vi "Process.vi"(8 "error in":errorcluster, 11 "Pump":refnum<class "Pump.lvclass">) -> (0 "error out":errorcluster, 3 "Pump out":refnum<class "Pump.lvclass">)   [LabVIEW 2014, in "Pump.lvclass"]
doc: "JKI State Machine Objects (SMO) 1.4.0.57\nJKI - JKI\nCopyright (c) 2018, JKI"
uses:
  Pump.lvclass
  <vilib>/JKI/JKI SMO/SMO/Typedefs/Parent Call--Enum.ctl
  Pump.lvclass/Pump.ctl
  Pump State - cluster.ctl
  <vilib>/addons/control/pid/pid.llb/PID Advanced (DBL).vi
  <vilib>/JKI/JKI SMO/SMO/SMO.lvclass
  <vilib>/addons/control/pid/NI_PID_pid.lvlib
panel:
  out "Pump State":T1(graph)
  # "For instructions on how to use the JKI State Machine Objects, examples and video tutorials, visit:\nhttp://jki.net/state-machine-objects/\n\nJKI State Machine Objects™\nhttp://jki.net/state-machine-objects/\nCopyright (C) 2005-2015, JKI <info@jki.net>\nALL RIGHTS RESERVED"
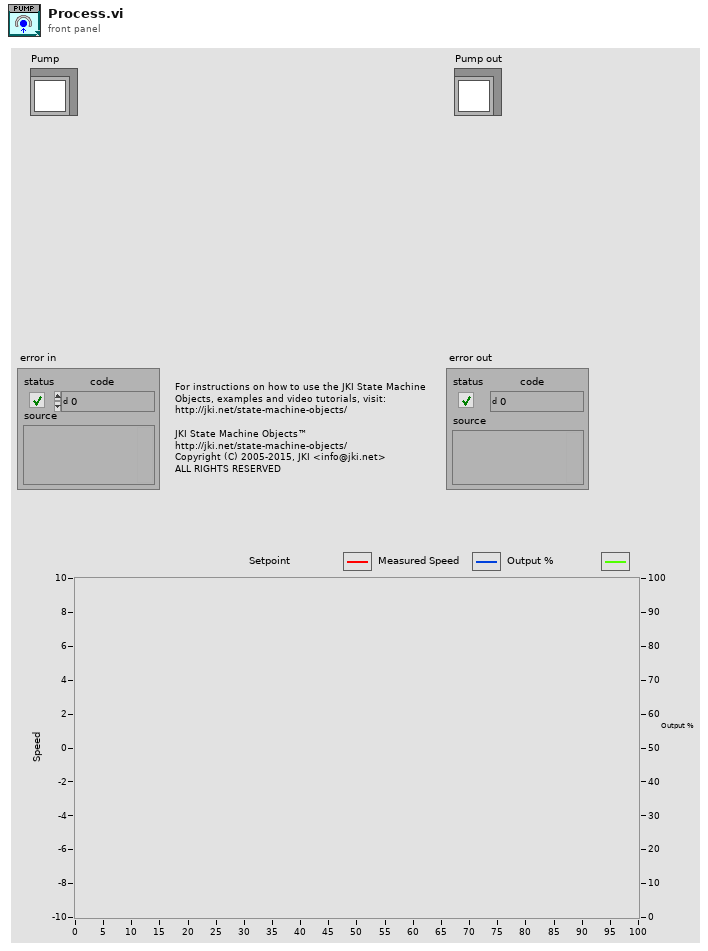
[diagram p1: front panel]
types:
  T1 = typedef "Pump.lvclass/Pump State - cluster.ctl" = cluster{"Pump Setpoint":dbl, "Pump Speed":dbl, "Output %":dbl}
  T2 = typedef "SMO.lvclass/Parent Call--Enum.ctl" = enum16{"Allows parent to run", "Does not request parent to run"}
  T3 = enum32{"invalid app kind", "Development System", "Run Time System", "Student Edition", "Embedded LabVIEW", "Evaluation", "Custom"}
  T4 = enum32{"Invalid", "Standard", "Closed", "Hidden", "Minimized", "Maximized"}
  T5 = cluster{"proportional gain (Kc)":dbl, "integral time (Ti, min)":dbl, "derivative time (Td, min)":dbl}
  T6 = typedef "Pump.lvclass/Parameters - cluster.ctl" = cluster{"Kc":dbl, "Ti":dbl, "Td":dbl, "Min Speed":dbl, "Max Speed":dbl}
  T7 = cluster{"Core":cluster{"Current VI Reference":refnum<vi>, "Close Panel on Exit?":bool, "error":errorcluster}, "Self Reference":refnum<class "Pump.lvclass">, "Parameters":T6, "Speed":dbl}
  T8 = cluster{"Current VI Reference":refnum<vi>, "Close Panel on Exit?":bool, "error":errorcluster}
  T9 = typedef "SMO.lvclass/Protected Events.ctl" = cluster{"StopProcesses":refnum<user-event>, "AbortProcesses":refnum<user-event>, "Config Changed":refnum<user-event>, "Dependency":refnum<user-event>}
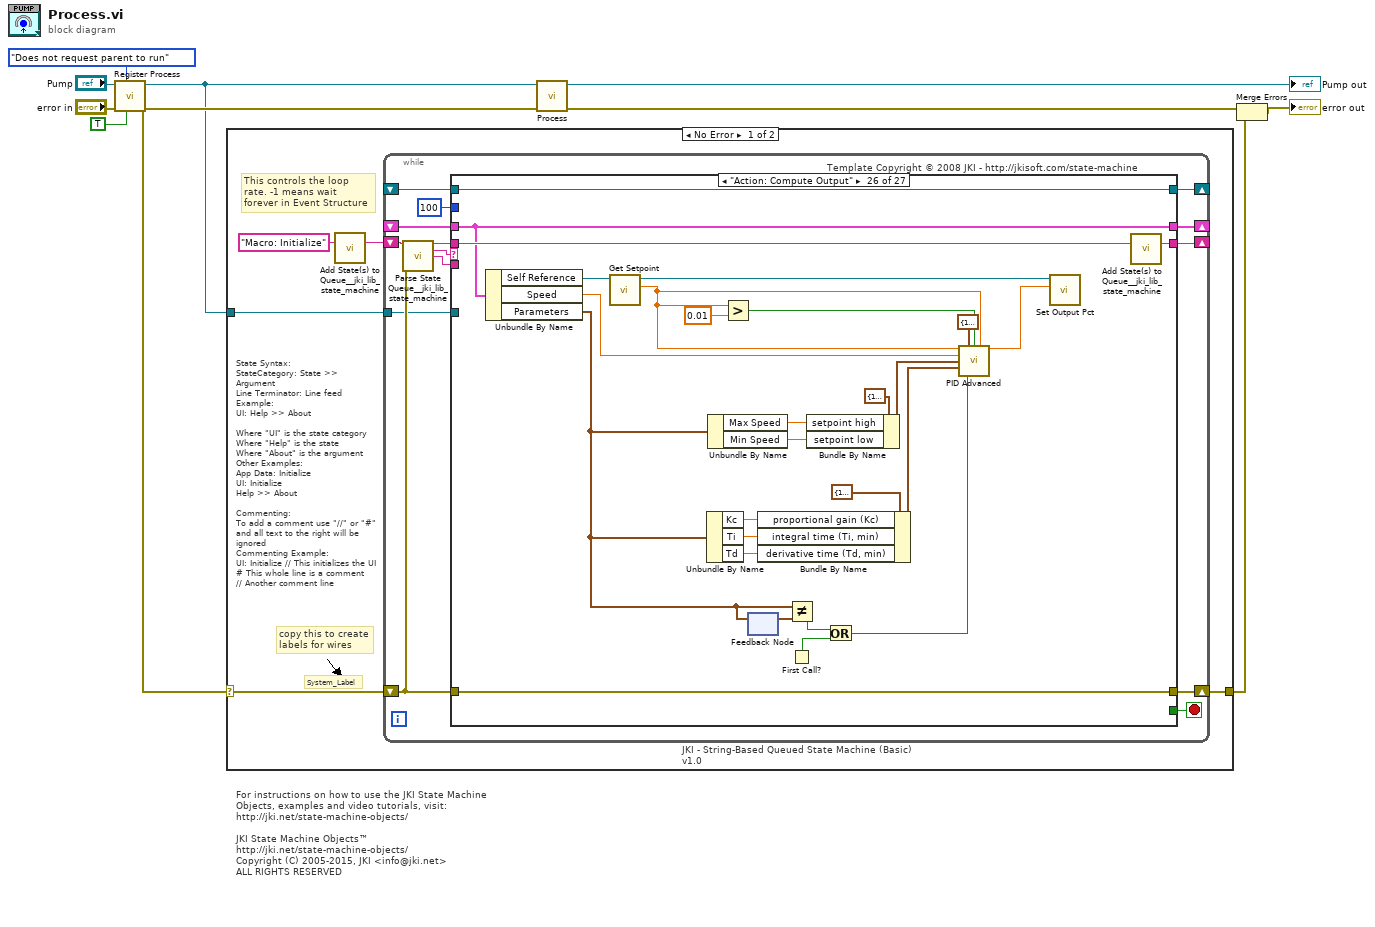
[diagram p0: block diagram]
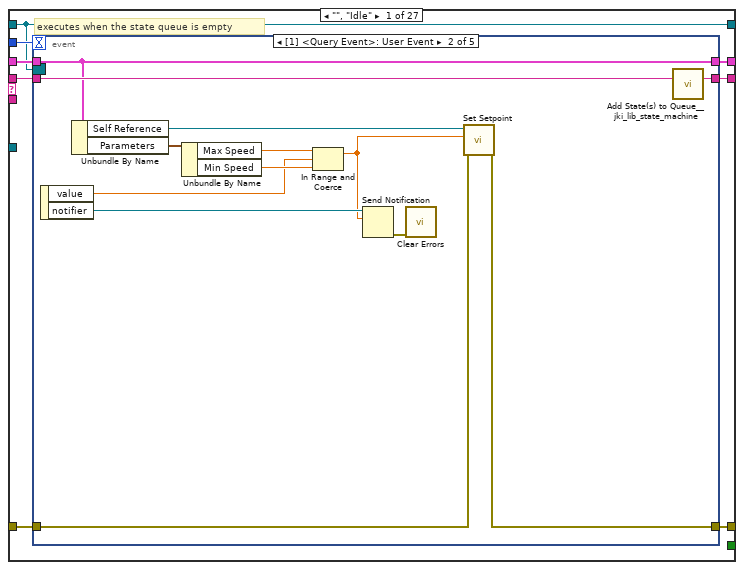
[diagram p2: hidden frame]
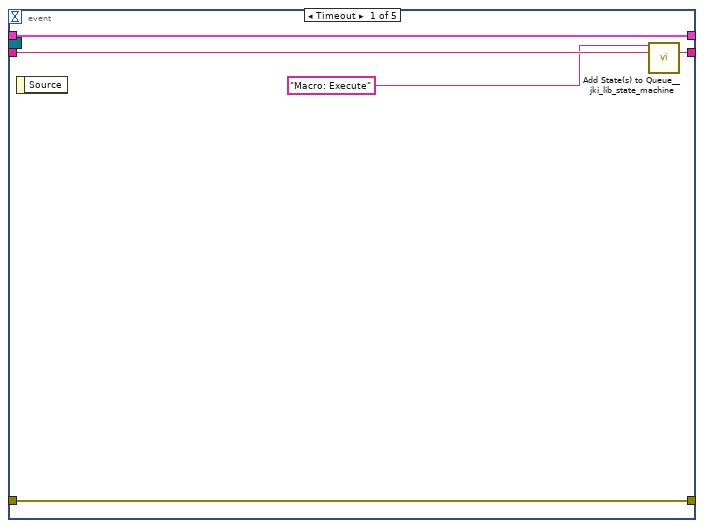
[diagram p3: hidden frame]
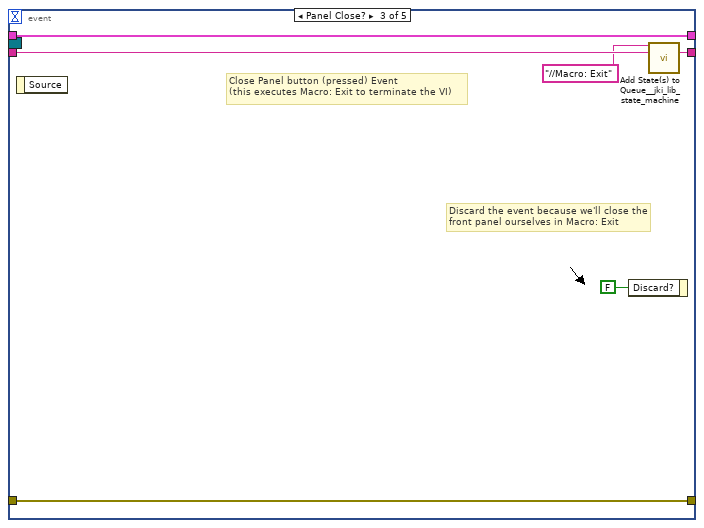
[diagram p4: hidden frame]
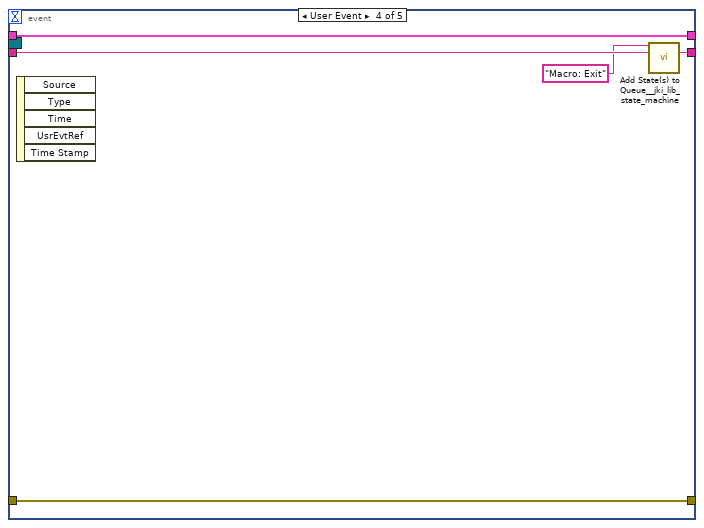
[diagram p5: hidden frame]
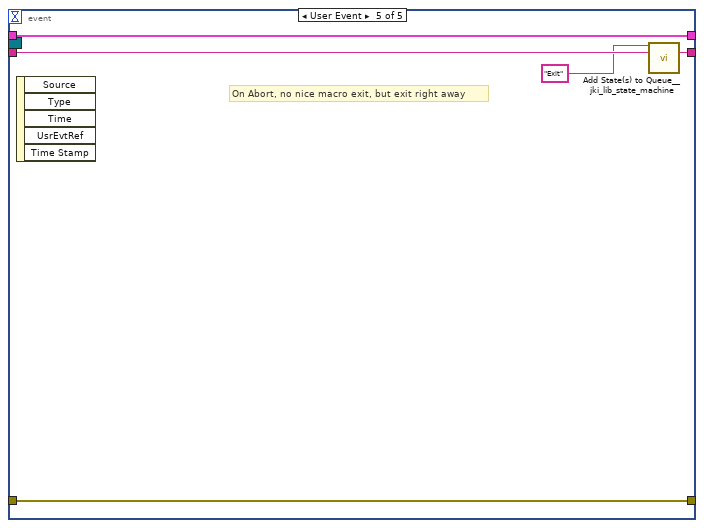
[diagram p6: hidden frame]
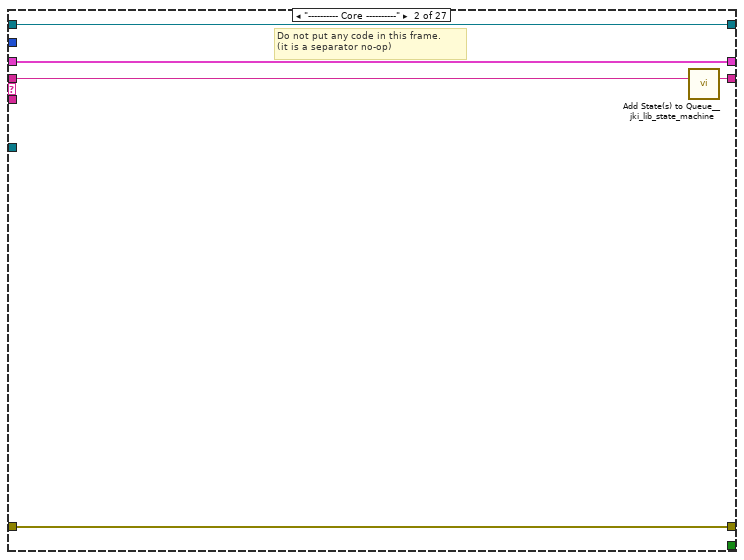
[diagram p7: hidden frame]
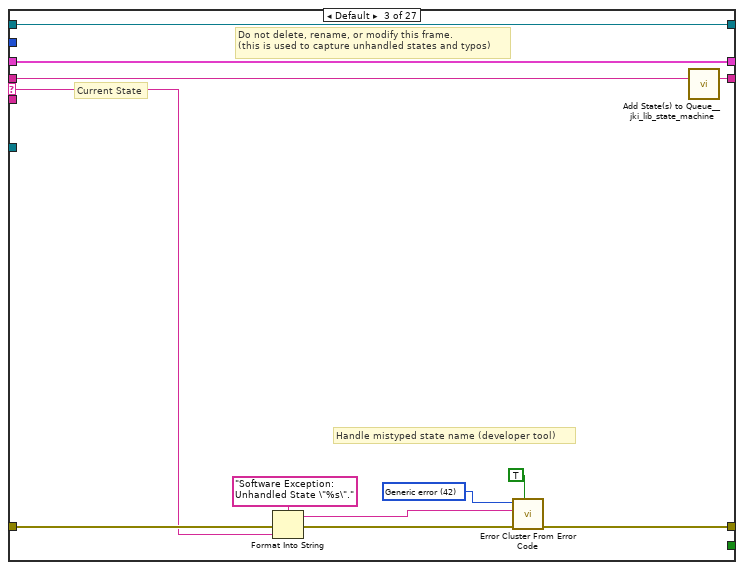
[diagram p8: hidden frame]
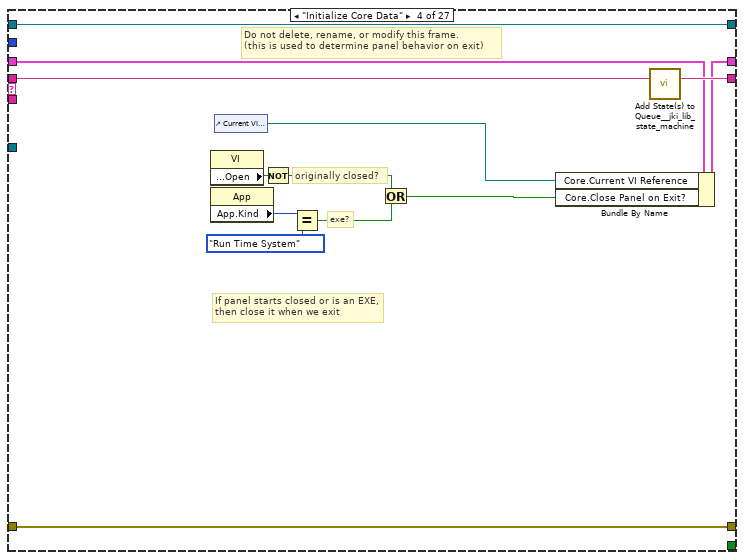
[diagram p9: hidden frame]
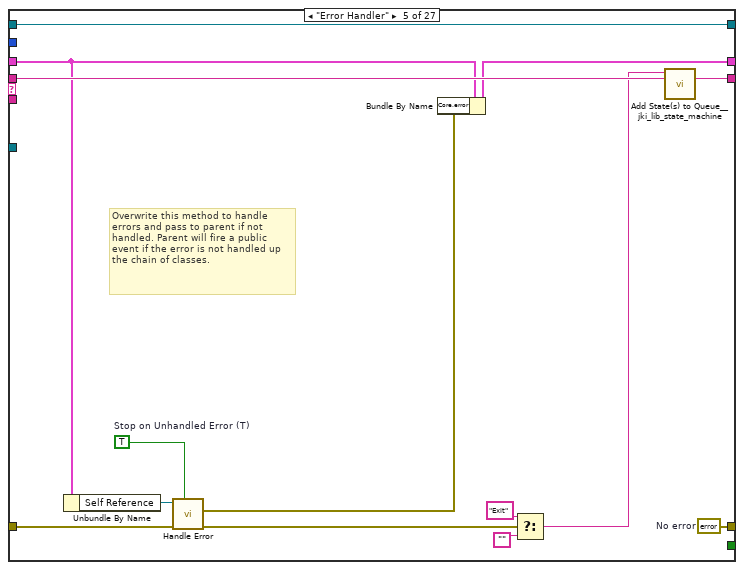
[diagram p10: hidden frame]
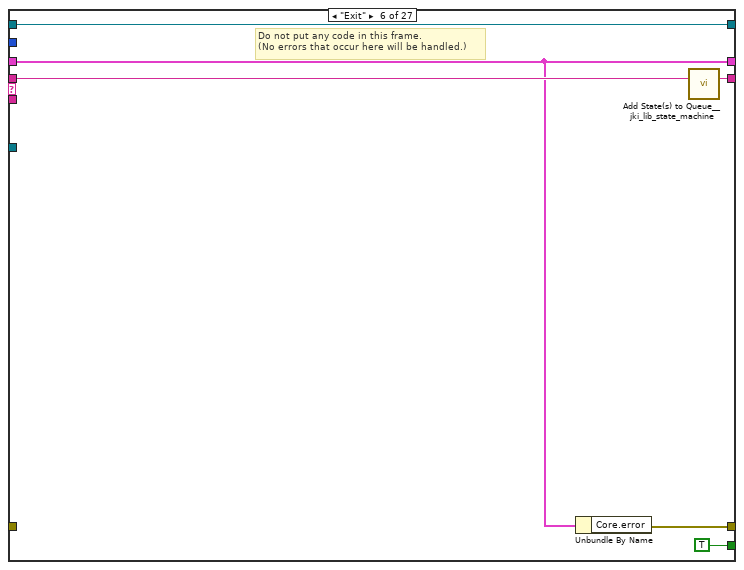
[diagram p11: hidden frame]
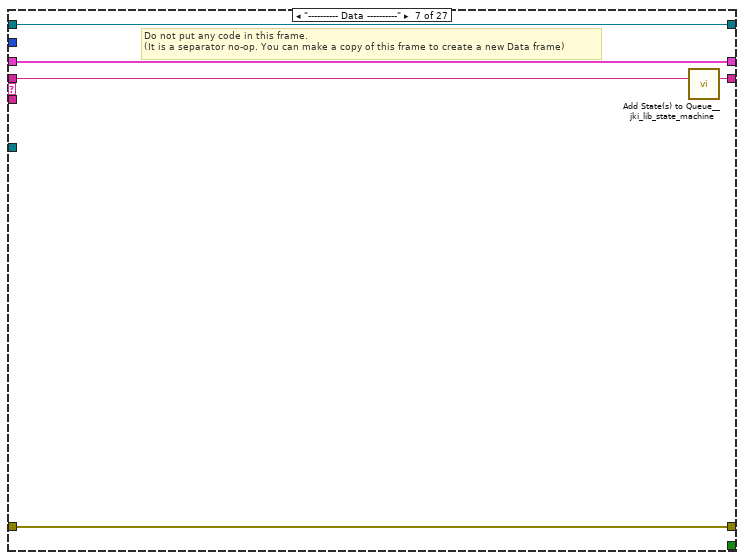
[diagram p12: hidden frame]
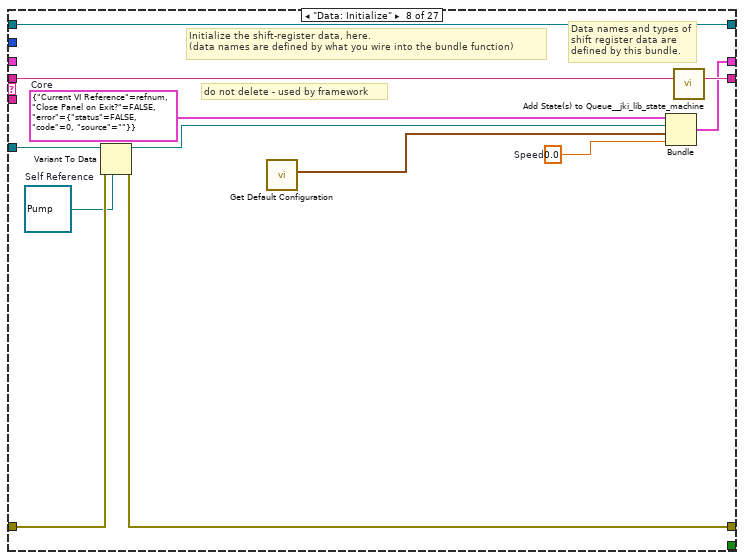
[diagram p13: hidden frame]
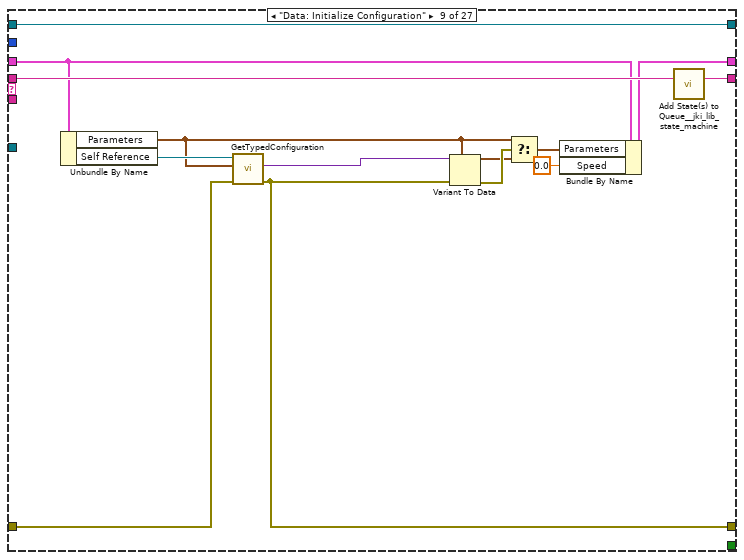
[diagram p14: hidden frame]
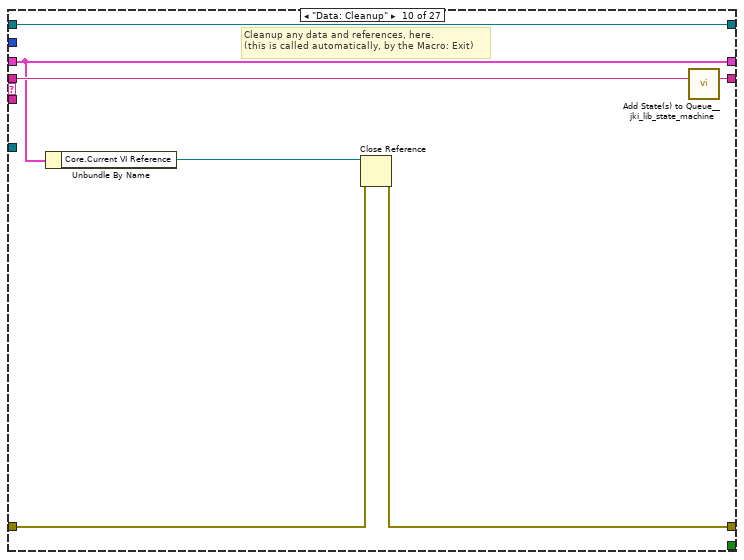
[diagram p15: hidden frame]
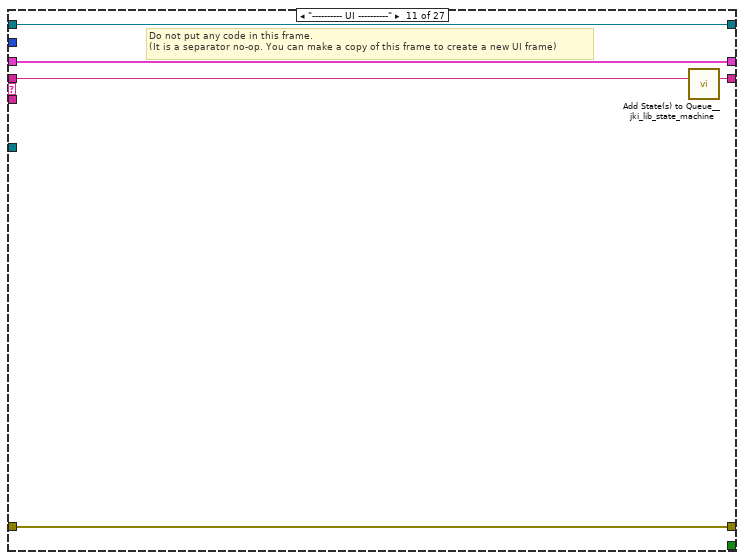
[diagram p16: hidden frame]
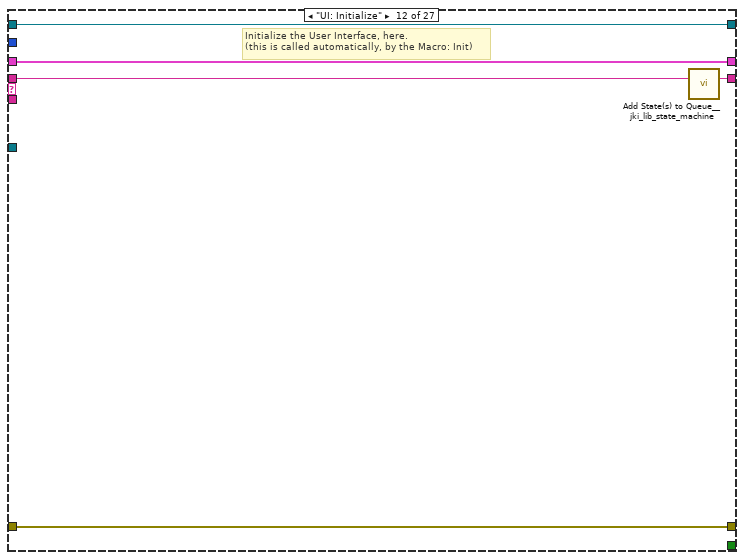
[diagram p17: hidden frame]
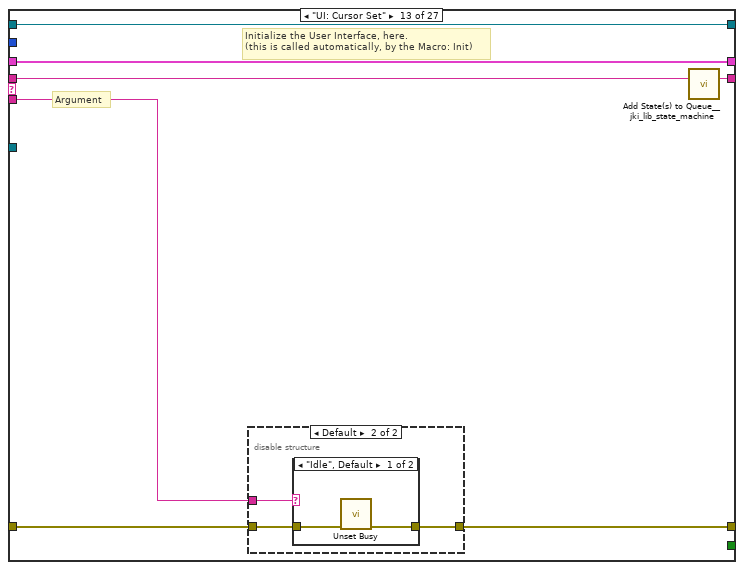
[diagram p18: hidden frame]
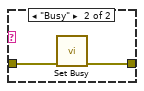
[diagram p20: hidden frame]
diagram:
  # "For instructions on how to use the JKI State Machine Objects, examples and video tutorials, visit:\nhttp://jki.net/state-machine-objects/\n\nJKI State Machine Objects™\nhttp://jki.net/state-machine-objects/\nCopyright (C) 2005-2015, JKI <info@jki.net>\nALL RIGHTS RESERVED"
  n1 = call <vilib>:"Register Process.vi"("Forces Self to Run (F)"=TRUE, "Parent Call"=Parent_Call--Enum."Does not request parent to run", "error in (no error)"="error in", "SMO"="Pump") -> ("error out"=w10:errorcluster, "SMO out"=w9:refnum<class "Pump.lvclass">)  [unwired: 6 in]
  n2 = case shown="No Error" w10 {
    selector: w10 -> [w12 w352]
    tunnel: w9 -> [w13 _]
    tunnel: [w11 w352] -> w7
    frame No Error {
      # "State Syntax:\nStateCategory: State >> Argument\nLine Terminator: Line feed\nExample:\nUI: Help >> About\n\nWhere \"UI\" is the state category\nWhere \"Help\" is the state\nWhere \"About\" is the argument\nOther Examples:\nApp Data: Initialize\nUI: Initialize\nHelp >> About\n\nCommenting:\nTo add a comment use \"//\" or \"#\" and all text to the right will be ignored\nCommenting Example:\nUI: Initialize // This initializes the UI\n# This whole line is a comment\n// Another comment line"
      # "copy this to create labels for wires"
      # "This controls the loop rate. -1 means wait forever in Event Structure"
      # "System_Label"
      n3 = call <vilib>:"Add State(s) to Queue__jki_lib_state_machine.vi"("State(s) in (\"\")"="Macro: Initialize") -> ("States Out"=w15:string)  [unwired: 14 in]
      n4 = while "JKI - String-Based Queued State Machine (Basic) v1.0" {
        shift-right: [w22] -> _
        shift-left: _ -> [w21]
        shift-right: [w25] -> w11
        shift-left: w12 -> [w19]
        shift-right: [w24] -> _
        shift-left: w15 -> [w26]
        tunnel: w13 -> [w18]
        shift-right: [w17] -> _
        shift-left: _ -> [w16]
        stop <- w23 stop-if-true
        # "Template Copyright © 2008 JKI - http://jkisoft.com/state-machine"
        n5 = call <vilib>:"Parse State Queue__jki_lib_state_machine.vi"("State Queue"=w26, "Error In (no error)"=w19) -> ("Remaining States"=w28:string, "Current State"=w29:string, "Arguments"=w27:string)  [unwired: 11 in]
        n6 = case shown="\"Action: Compute Output\"" w29 {
          selector: w29 -> [_ _ w78 _ _ _ _ _ _ _ _ _ _ _ _ _ _ _ _ _ _ _ _ _ _ _ _]
          tunnel: w28 -> [w37 w76 w82 w101 w115 w121 w126 w138 w152 w159 w164 w169 w176 w192 w224 w233 w239 w253 w258 w269 w274 w285 w291 w296 w306 w333 w351]
          tunnel: w27 -> [_ _ _ _ _ _ _ _ _ _ _ _ w170 w186 _ _ _ _ _ _ _ _ _ _ _ _ _]
          tunnel: w21 -> [w35 w73 w80 w92 w109 w117 w123 _ w149 w154 w161 w167 w174 w188 w221 w229 w235 w244 w255 w266 w271 w283 w289 w294 w303 w315 w348]
          tunnel: [w34 w74 w84 w98 w110 w116 w124 w134 w141 w155 w162 w166 w171 w189 w222 w231 w237 w251 w256 w260 w272 w280 w287 w292 w302 w330 w341] -> w25
          tunnel: w19 -> [w33 w74 w83 w98 w111 _ w124 w135 w142 w156 w162 w166 w172 w190 w222 w231 w237 w251 w256 w261 w272 w281 w287 w292 w298 w330 w342]
          tunnel: [w36 w75 w81 w100 w114 w120 w125 w137 w151 w158 w163 w168 w175 w191 w223 w232 w238 w252 w257 w268 w273 w284 w290 w295 w305 w332 w350] -> w24
          tunnel: [_ _ _ _ _ TRUE _ _ _ _ _ _ _ _ _ _ _ _ _ _ _ _ _ _ _ _ _] -> w23
          tunnel: [w32 w73 w80 w99 w108 w117 w123 w136 w148 w154 w161 w167 w174 w188 w221 w229 w235 w244 w255 w266 w271 w283 w289 w294 w303 w315 w347] -> w22
          tunnel: 100 ("Timeout") -> [w31 _ _ _ _ _ _ _ _ _ _ _ _ _ _ _ _ _ _ _ _ _ _ _ _ _ _]
          tunnel: w18 -> [_ _ _ _ _ _ _ w133 _ _ _ _ _ _ _ _ _ _ _ _ _ _ _ _ _ _ _]
          tunnel: [w30 w72 w77 w89 w113 w118 w122 w131 w150 w153 w160 w165 w173 w185 w220 w230 w236 w245 w254 w267 w270 w275 w288 w293 w304 w331 w349] -> w17
          tunnel: w16 -> [w30 w72 w77 w89 w113 w118 w122 w131 w150 w153 w160 w165 w173 w185 w220 w230 w236 w245 w254 w267 w270 _ w288 w293 w304 w331 w349]
          frame "", "Idle" {
            # "executes when the state queue is empty"
            n7 = event shown="[1] <Query Event>: User Event" {
              selector: w30 -> [_ _ _ _ _]
              dyn-events: _ -> [_ _ _ _ _]
              timeout: w31 -> [_ _ _ _ _]
              tunnel: w37 -> [w42 w55 w61 w66 w71]
              tunnel: [w41 w54 w60 w65 w70] -> w36
              tunnel: w35 -> [w38 w45 w58 w63 w68]
              tunnel: [w40 w43 w59 w64 w69] -> w34
              tunnel: w33 -> [w40 w44 w59 w64 w69]
              tunnel: [w38 w45 w58 w63 w68] -> w32
              event Timeout {
                n8 = event-data() -> ()  [unwired: 1 in, 1 out]
                n9 = call <vilib>:"Add State(s) to Queue__jki_lib_state_machine.vi"("State(s) in Front (\"\")"="Macro: Execute", "State(s) in (\"\")"=w42) -> ("States Out"=w41:string)  [unwired: 13 in]
              }
              event User Event {
                n10 = event-data() -> ("value"=w48:dbl, "notifier"=w52:refnum<notifier>)  [unwired: 1 in]
                n11 = Unbundle By Name(w45) -> ("Self Reference"=w47:refnum<class "Pump.lvclass">, "Parameters"=w51:T6)
                n12 = Unbundle By Name(w51) -> ("Max Speed"=w50:dbl, "Min Speed"=w49:dbl)
                n13 = In Range and Coerce(upper limit=w50, x=w48, lower limit=w49) -> (coerced(x)=w46:dbl)  [unwired: 1 out]
                n14 = Send Notification(notification=w46, notifier=w52) -> (error out=w53:errorcluster)  [unwired: 1 in, 1 out]
                n15 = call <vilib>:"Clear Errors.vi"("error in (no error)"=w53) -> ()  [unwired: 5 in, 2 out]
                n16 = call "Set Setpoint.vi"("error in (no error)"=w44, "Setpoint"=w46, "Pump in"=w47) -> ("error out"=w43:errorcluster)  [unwired: 7 in, 1 out]
                n17 = call <vilib>:"Add State(s) to Queue__jki_lib_state_machine.vi"("State(s) in (\"\")"=w55) -> ("States Out"=w54:string)  [unwired: 14 in]
              }
              event Panel Close? {
                # "Discard the event because we'll close the front panel ourselves in Macro: Exit"
                # "Close Panel button (pressed) Event\n(this executes Macro: Exit to terminate the VI)"
                n18 = event-data() -> ()  [unwired: 1 in, 1 out]
                n19 = event-data("Discard?"=FALSE) -> ()  [unwired: 1 in, 1 out]
                n20 = call <vilib>:"Add State(s) to Queue__jki_lib_state_machine.vi"("State(s) in Front (\"\")"="//Macro: Exit", "State(s) in (\"\")"=w61) -> ("States Out"=w60:string)  [unwired: 13 in]
              }
              event User Event {
                n21 = event-data() -> ()  [unwired: 1 in, 5 out]
                n22 = call <vilib>:"Add State(s) to Queue__jki_lib_state_machine.vi"("State(s) in Front (\"\")"="Macro: Exit", "State(s) in (\"\")"=w66) -> ("States Out"=w65:string)  [unwired: 13 in]
              }
              event User Event {
                # "On Abort, no nice macro exit, but exit right away"
                n23 = event-data() -> ()  [unwired: 1 in, 5 out]
                n24 = call <vilib>:"Add State(s) to Queue__jki_lib_state_machine.vi"("State(s) in Front (\"\")"="Exit", "State(s) in (\"\")"=w71) -> ("States Out"=w70:string)  [unwired: 13 in]
              }
            }
          }
          frame "---------- Core ----------" {
            # "Do not put any code in this frame.\n(it is a separator no-op)"
            n25 = call <vilib>:"Add State(s) to Queue__jki_lib_state_machine.vi"("State(s) in (\"\")"=w76) -> ("States Out"=w75:string)  [unwired: 14 in]
          }
          frame Default {
            w87 = 42 items=["No error", "Argument error", "Memory is full", "Out of zone", "End of file", "File already open", "Generic file I/O error", "File not found", "File permission error", "Disk is full", "Duplicate path", "Too many files open", "System feature not enabled", "Resource file not found", "Cannot add resource", "Resource not found", "Image not found", "Image memory error", "Pen does not exist", "Config type invalid", "Config token not found", "Config parse error", "Config memory error", "Bad external code format", "Bad external code offset", "External code not present", "Null window", "Destroy window error", "Null menu", "Print aborted", "Bad print record", "Print driver error", "Windows error during printing", "Memory error during printing", "Print dialog error", "Generic print error", "Invalid device refnum", "Device not found", "Device parameter error", "Device unit error", "Cannot open device", "Device call aborted", "Generic error", "Cancelled by user", "Object ID too low", "Object ID too high", "Object not in heap", "Unknown heap", "Unknown object (invalid DefProc)", "Unknown object (DefProc not in table)", "Message out of range", "Invalid (null) method", "Unknown message", "Manager call not supported", "Bad address", "Network operation in progress", "Network operation timed out", "Connection is busy", "Network attribute not supported", "Network error", "Address in use", "System out of memory", "Connection aborted", "Connection refused", "Not connected", "Already connected", "Connection closed", "Initialization error (interapplication manager)", "Bad occurrence", "Wait on unbound occurrence handler", "Occurrence queue overflow", "Datalog type conflict", "Unused", "Unrecognized type (interapplication manager)", "Memory corrupt", "Failed to make temporary DLL", "Old CIN version", "Drag socket not found", "Failed to load drop-object", "Failed to register OLE object", "Failed to release OLE object", "Format specifier type mismatch", "Unknown format specifier", "Too few format specifiers", "Too many format specifiers", "Scan failed", "Newer CIN version", "Error converting to variant", "Runtime menu error", "Password tampered", "Variant attribute not found", "Incompatible variant data type", "Event data is not available", "Event Store is not present", "Occurrence is not found", "Event Queue is not created", "Event info is not available", "Refnum passed is NULL", "Error retrieving Class GUID", "Error retrieving CoClass GUID", "Error retrieving TypeLib GUID.", "Bad built application magic bytes.", "Specific driver is different from the specific driver associated with the Logical Name.", "There is no session opened to the class driver.", "Max Error", "MAX - Error with config objects", "MAX - Error loading configuration", "MAX - Group not supported"]
            # "Current State"
            # "Do not delete, rename, or modify this frame.\n(this is used to capture unhandled states and typos)"
            # "Handle mistyped state name (developer tool)"
            n26 = Format Into String(format string="Software Exception: Unhandled State \"%s\"." ("message"), error in=w83, w78) -> (resulting string=w86:string, error out=w85:errorcluster)  [unwired: 1 in]
            n27 = call <vilib>:"Error Cluster From Error Code.vi"("show call chain? (False)"=TRUE, "error in (no error)"=w85, "error message (\"\")"=w86, "error code (0)"=w87) -> ("error out"=w84:errorcluster)  [unwired: 5 in]
            n28 = call <vilib>:"Add State(s) to Queue__jki_lib_state_machine.vi"("State(s) in (\"\")"=w82) -> ("States Out"=w81:string)  [unwired: 14 in]
          }
          frame "Initialize Core Data" {
            # "Do not delete, rename, or modify this frame.\n(this is used to determine panel behavior on exit)"
            # "originally closed?"
            # "exe?"
            # "If panel starts closed or is an EXE, then close it when we exit"
            n29 = property class="VI"() -> ("Front Panel.Open"=w97:bool)  [unwired: 2 in, 2 out]
            n30 = property class="App"() -> ("App.Kind"=w96:T3)  [unwired: 2 in, 2 out]
            n31 = control-ref of="Current VI Reference"() -> (w90:refnum<vi>)
            n32 = Not(x=w97) -> (.not. x?=w94:bool)
            n33 = Equal?(x=w96, y=T3."Run Time System" ("Application:Kind")) -> (x = y?=w93:bool)
            n34 = Or(x=w94, y=w93) -> (x .or. y?=w91:bool)
            n35 = Bundle By Name(cluster=w92, "Core.Current VI Reference"=w90, "Core.Close Panel on Exit?"=w91) -> (w99:T7)
            n36 = call <vilib>:"Add State(s) to Queue__jki_lib_state_machine.vi"("State(s) in (\"\")"=w101) -> ("States Out"=w100:string)  [unwired: 14 in]
          }
          frame "Error Handler" {
            w102 = TRUE  # Stop on Unhandled Error (T)
            w110 = errorcluster {"status"=FALSE, "code"=0, "source"=""}  # No error
            # "Overwrite this method to handle errors and pass to parent if not handled. Parent will fire a public event if the error is not handled up the chain of classes."
            n37 = Unbundle By Name(w109) -> ("Self Reference"=w112:refnum<class "Pump.lvclass">)
            n38 = call-dynamic "Handle Error.vi"("Stop on Unhandled Error (T)"=w102, "error in"=w111, "SMO"=w112) -> ("handling error"=w103:errorcluster, "Unhandled error"=w106:errorcluster)  [unwired: 6 in, 1 out]
            n39 = Bundle By Name(cluster=w109, "Core.error"=w106) -> (w108:T7)
            n40 = Select(t="Exit", s=w103, f="") -> (s? t:f=w107:string)
            n41 = call <vilib>:"Add State(s) to Queue__jki_lib_state_machine.vi"("State(s) in Front (\"\")"=w107, "State(s) in (\"\")"=w115) -> ("States Out"=w114:string)  [unwired: 13 in]
          }
          frame "Exit" {
            # "Do not put any code in this frame.\n(No errors that occur here will be handled.)"
            n42 = Unbundle By Name(w117) -> ("Core.error"=w116:errorcluster)
            n43 = call <vilib>:"Add State(s) to Queue__jki_lib_state_machine.vi"("State(s) in (\"\")"=w121) -> ("States Out"=w120:string)  [unwired: 14 in]
          }
          frame "---------- Data ----------" {
            # "Do not put any code in this frame.\n(It is a separator no-op. You can make a copy of this frame to create a new Data frame)"
            n44 = call <vilib>:"Add State(s) to Queue__jki_lib_state_machine.vi"("State(s) in (\"\")"=w126) -> ("States Out"=w125:string)  [unwired: 14 in]
          }
          frame "Data: Initialize" {
            w127 = 0.0  # Speed
            w129 = refnum<class "Pump.lvclass"> refnum  # Self Reference
            w130 = T8 {"Current VI Reference"=refnum, "Close Panel on Exit?"=FALSE, "error"={"status"=FALSE, "code"=0, "source"=""}}  # Core
            # "do not delete - used by framework"
            # "Data names and types of shift register data are defined by this bundle."
            # "Initialize the shift-register data, here.\n(data names are defined by what you wire into the bundle function)"
            n45 = Variant To Data(error in=w135, type=w129, Variant=w133) -> (data=w132:refnum<class "Pump.lvclass">, error out=w134:errorcluster)
            n46 = call "Get Default Configuration.vi"() -> ("Parameters"=w128:T6)  [unwired: 11 in]
            n47 = Bundle("Core"=w130, "Self Reference"=w132, "Parameters"=w128, "Speed"=w127) -> (w136:T7)  [unwired: 1 in]
            n48 = call <vilib>:"Add State(s) to Queue__jki_lib_state_machine.vi"("State(s) in (\"\")"=w138) -> ("States Out"=w137:string)  [unwired: 14 in]
          }
          frame "Data: Initialize Configuration" {
            n49 = Unbundle By Name(w149) -> ("Parameters"=w140:T6, "Self Reference"=w144:refnum<class "Pump.lvclass">)
            n50 = call <vilib>:"GetTypedConfiguration.vi"("error in (no error)"=w142, "Default value"=w140, "SMO"=w144) -> ("error out"=w141:errorcluster, "Variant"=w143:variant)  [unwired: 4 in, 3 out]
            n51 = Variant To Data(error in=w141, type=w140, Variant=w143) -> (data=w146:T6, error out=w147:errorcluster)
            n52 = Select(t=w140, s=w147, f=w146) -> (s? t:f=w145:T6)
            n53 = Bundle By Name(cluster=w149, "Parameters"=w145, "Speed"=0.0 ("Setpoint")) -> (w148:T7)
            n54 = call <vilib>:"Add State(s) to Queue__jki_lib_state_machine.vi"("State(s) in (\"\")"=w152) -> ("States Out"=w151:string)  [unwired: 14 in]
          }
          frame "Data: Cleanup" {
            # "Cleanup any data and references, here.\n(this is called automatically, by the Macro: Exit)"
            n55 = Unbundle By Name(w154) -> ("Core.Current VI Reference"=w157:refnum<vi>)
            n56 = Close Reference(reference=w157, error in (no error)=w156) -> (error out=w155:errorcluster)
            n57 = call <vilib>:"Add State(s) to Queue__jki_lib_state_machine.vi"("State(s) in (\"\")"=w159) -> ("States Out"=w158:string)  [unwired: 14 in]
          }
          frame "---------- UI ----------" {
            # "Do not put any code in this frame.\n(It is a separator no-op. You can make a copy of this frame to create a new UI frame)"
            n58 = call <vilib>:"Add State(s) to Queue__jki_lib_state_machine.vi"("State(s) in (\"\")"=w164) -> ("States Out"=w163:string)  [unwired: 14 in]
          }
          frame "UI: Initialize" {
            # "Initialize the User Interface, here.\n(this is called automatically, by the Macro: Init)"
            n59 = call <vilib>:"Add State(s) to Queue__jki_lib_state_machine.vi"("State(s) in (\"\")"=w169) -> ("States Out"=w168:string)  [unwired: 14 in]
          }
          frame "UI: Cursor Set" {
            # "Argument"
            # "Initialize the User Interface, here.\n(this is called automatically, by the Macro: Init)"
            n60 = disable-structure shown="Default" {
              disable-tunnel: w172 -> [w177 w180]
              disable-tunnel: [w177 w179] -> w171
              disable-tunnel: w170 -> [_ w178]
              frame condition #0 {
              }
              frame condition #1 (active) {
                n61 = case shown="\"Idle\", Default" w178 {
                  tunnel: w180 -> [w182 w184]
                  tunnel: [w181 w183] -> w179
                  frame "Idle", Default {
                    n62 = call <vilib>:"Unset Busy.vi"("error in (no error)"=w182) -> ("error out"=w181:errorcluster)  [unwired: 10 in]
                  }
                  frame "Busy" {
                    n63 = call <vilib>:"Set Busy.vi"("error in (no error)"=w184) -> ("error out"=w183:errorcluster)  [unwired: 9 in, 1 out]
                  }
                }
              }
            }
            n64 = call <vilib>:"Add State(s) to Queue__jki_lib_state_machine.vi"("State(s) in (\"\")"=w176) -> ("States Out"=w175:string)  [unwired: 14 in]
          }
          frame "UI: Front Panel State" {
            # "Argument"
            # "Set Front Panel Open or Closed\n(Usage: \"UI: Front Panel State >> Open|Close\")"
            n65 = Unbundle By Name(w188) -> ("Core.Current VI Reference"=w187:refnum<vi>)
            n66 = disable-structure shown="Default" {
              disable-tunnel: w190 -> [w196 w219]
              disable-tunnel: [w195 w219] -> w189
              disable-tunnel: w187 -> [w194 _]
              disable-tunnel: w186 -> [w193 _]
              frame condition #0 (active) {
                n67 = case shown="\"Close\"" w193 {
                  tunnel: w196 -> [w200 w213]
                  tunnel: [w202 w214] -> w195
                  tunnel: w194 -> [w201 w211]
                  frame "Open", Default {
                    n68 = property class="VI"(reference=w201, error in=w200) -> (reference out=w198:refnum<vi>, error out=w199:errorcluster, "FP.State"=w197:T4)
                    n69 = case shown="\"Closed\"" w197 {
                      tunnel: [w205 w208] -> w202
                      tunnel: w199 -> [w204 w208]
                      tunnel: w198 -> [w203 _]
                      frame "Closed" {
                        n70 = invoke class="VI" method="FP.Open"(reference=w203, error in=w204, "Activate"=TRUE, "State"=T4."Standard") -> (error out=w205:errorcluster)  [unwired: 1 in, 4 out]
                      }
                      frame Default {
                      }
                    }
                  }
                  frame "Close" {
                    n71 = property class="VI"(reference=w211, error in=w213) -> (reference out=w210:refnum<vi>, error out=w212:errorcluster, "FP.State"=w209:T4)
                    n72 = case shown="Default" w209 {
                      tunnel: [w215 w218] -> w214
                      tunnel: w212 -> [w215 w217]
                      tunnel: w210 -> [_ w216]
                      frame "Invalid", "Closed" {
                      }
                      frame Default {
                        n73 = invoke class="VI" method="FP.Close"(reference=w216, error in=w217) -> (error out=w218:errorcluster)  [unwired: 1 in, 2 out]
                      }
                    }
                  }
                }
              }
              frame condition #1 {
              }
            }
            n74 = call <vilib>:"Add State(s) to Queue__jki_lib_state_machine.vi"("State(s) in (\"\")"=w192) -> ("States Out"=w191:string)  [unwired: 14 in]
          }
          frame "---------- Macro ----------" {
            # "Do not put any code in this frame.\n(It is a separator no-op. You can make a copy of this frame to create a new Macro frame)"
            n75 = call <vilib>:"Add State(s) to Queue__jki_lib_state_machine.vi"("State(s) in (\"\")"=w224) -> ("States Out"=w223:string)  [unwired: 14 in]
          }
          frame "Macro: Initialize" {
            w227 = "//UI: Initialize\n//UI: Front Panel State >> Open"  # //UI: Initialize //UI: Front Panel State >> Open
            # "Initialization Macro\n(This is called once, when the VI starts)"
            n76 = call <vilib>:"Add State(s) to Queue__jki_lib_state_machine.vi"("State(s) in Front (\"\")"="Data: Initialize\nInitialize Core Data\nEvents: Register\nData: Initialize Configuration", "State(s) in (\"\")"="Process: Sync", "State(s) at Back (\"\")"=w227) -> ("States Out"=w226:string)  [unwired: 12 in]
            n77 = call <vilib>:"Add State(s) to Queue__jki_lib_state_machine.vi"("State(s) in Front (\"\")"=w226, "State(s) in (\"\")"=w233) -> ("States Out"=w232:string)  [unwired: 13 in]
          }
          frame "Macro: Execute" {
            n78 = call <vilib>:"Add State(s) to Queue__jki_lib_state_machine.vi"("State(s) in Front (\"\")"="Action: Read Speed\nAction: Compute Output\nAction: Control Pump", "State(s) in (\"\")"=w239) -> ("States Out"=w238:string)  [unwired: 13 in]
          }
          frame "Macro: Exit" {
            # "Exit Macro\n(This is called once, when the VI exits)"
            n79 = Unbundle By Name(w244) -> ("Core.Close Panel on Exit?"=w250:bool)
            n80 = Select(t="UI: Front Panel State >> Close", s=w250, f="") -> (s? t:f=w247:string)
            n81 = call <vilib>:"Add State(s) to Queue__jki_lib_state_machine.vi"("State(s) in Front (\"\")"="Data: Cleanup\nEvents: Unregister", "State(s) in (\"\")"="Process: Sync", "State(s) at Back (\"\")"="Exit") -> ("States Out"=w241:string)  [unwired: 12 in]
            n82 = call <vilib>:"Add State(s) to Queue__jki_lib_state_machine.vi"("State(s) in (\"\")"=w247, "State(s) at Back (\"\")"=w241) -> ("States Out"=w246:string)  [unwired: 13 in]
            n83 = call <vilib>:"Add State(s) to Queue__jki_lib_state_machine.vi"("State(s) in Front (\"\")"=w246, "State(s) in (\"\")"=w253) -> ("States Out"=w252:string)  [unwired: 13 in]
          }
          frame "---------- Process ----------" {
            # "Template Separator\n(You can make a copy of, or modify, this frame)"
            n84 = call <vilib>:"Add State(s) to Queue__jki_lib_state_machine.vi"("State(s) in (\"\")"=w258) -> ("States Out"=w257:string)  [unwired: 14 in]
          }
          frame "Process: Sync" {
            n85 = Unbundle By Name(w266) -> ("Self Reference"=w262:refnum<class "Pump.lvclass">)
            n86 = call <vilib>:"WaitOnProcessSync.vi"("error in (no error)"=w261, "SMO"=w262) -> ("error out"=w260:errorcluster, "Don't run?"=w265:bool)  [unwired: 7 in, 1 out]
            n87 = Select(t="Data: Cleanup\nEvents: Unregister\nExit", s=w265, f="") -> (s? t:f=w259:string)
            n88 = call <vilib>:"Add State(s) to Queue__jki_lib_state_machine.vi"("State(s) in Front (\"\")"=w259, "State(s) in (\"\")"=w269) -> ("States Out"=w268:string)  [unwired: 13 in]
          }
          frame "---------- Events ----------" {
            # "Template Separator\n(You can make a copy of, or modify, this frame)"
            n89 = call <vilib>:"Add State(s) to Queue__jki_lib_state_machine.vi"("State(s) in (\"\")"=w274) -> ("States Out"=w273:string)  [unwired: 14 in]
          }
          frame "Events: Register" {
            # "Expand to add\nmore events"
            n90 = Unbundle By Name(w283) -> ("Self Reference"=w277:refnum<class "Pump.lvclass">)
            n91 = call <vilib>:"GetProtectedEvents.vi"("SMO"=w277) -> ("error out"=w278:errorcluster, "SMO Protected Events"=w282:T9)  [unwired: 8 in, 1 out]
            n92 = Unbundle By Name(w277) -> ("Query Event"=w276:refnum<user-event>)
            n93 = register-events(w282, w276) -> (reference out=w275:refnum<event-registration>, error out=w279:errorcluster)  [unwired: 2 in]
            n94 = Merge Errors(w281, w279, w278) -> (w280:errorcluster)
            n95 = call <vilib>:"Add State(s) to Queue__jki_lib_state_machine.vi"("State(s) in (\"\")"=w285) -> ("States Out"=w284:string)  [unwired: 14 in]
          }
          frame "Events: Unregister" {
            n96 = Unregister For Events(event registration refnum=w288, error in=w287) -> (error out=w286:errorcluster)
            n97 = call <vilib>:"Clear Errors.vi"("error in (no error)"=w286) -> ()  [unwired: 5 in, 2 out]
            n98 = call <vilib>:"Add State(s) to Queue__jki_lib_state_machine.vi"("State(s) in (\"\")"=w291) -> ("States Out"=w290:string)  [unwired: 14 in]
          }
          frame "---------- Action ----------" {
            n99 = call <vilib>:"Add State(s) to Queue__jki_lib_state_machine.vi"("State(s) in (\"\")"=w296) -> ("States Out"=w295:string)  [unwired: 14 in]
          }
          frame "Action: Control Pump" {
            n100 = Unbundle By Name(w303) -> ("Self Reference"=w301:refnum<class "Pump.lvclass">)
            n101 = call-dynamic "Get Output Pct.vi"("error in (no error)"=w298, "Pump in"=w301) -> ("error out"=w297:errorcluster, "Output %"=w299:dbl, "Pump out"=w300:refnum<class "Pump.lvclass">)  [unwired: 7 in]
            n102 = call-dynamic "writePumpSpeed.vi"("error in (no error)"=w297, "Output %"=w299, "Pump in"=w300) -> ("error out"=w302:errorcluster)  [unwired: 7 in, 1 out]
            n103 = call <vilib>:"Add State(s) to Queue__jki_lib_state_machine.vi"("State(s) in (\"\")"=w306) -> ("States Out"=w305:string)  [unwired: 14 in]
          }
          frame "Action: Compute Output" {
            n104 = Unbundle By Name(w315) -> ("Self Reference"=w329:refnum<class "Pump.lvclass">, "Speed"=w328:dbl, "Parameters"=w310:T6)
            n105 = call "Get Setpoint.vi"("Pump in"=w329) -> ("Pump Setpoint"=w308:dbl, "Pump out"=w317:refnum<class "Pump.lvclass">)  [unwired: 8 in, 1 out]
            n106 = Unbundle By Name(w310) -> ("Kc"=w321:dbl, "Ti"=w320:dbl, "Td"=w319:dbl)
            n107 = Unbundle By Name(w310) -> ("Max Speed"=w312:dbl, "Min Speed"=w313:dbl)
            n108 = Greater?(x=w308, y=0.01) -> (0:w309:bool)
            n109 = feedback #1() -> (w326:T6)  [unwired: 1 in]
            n110 = feedback-in #1(w310) -> ()
            n111 = Bundle By Name(cluster=T5 {"proportional gain (Kc)"=1.0, "integral time (Ti, min)"=0.01, "derivative time (Td, min)"=0.0} ("PID gains"), "proportional gain (Kc)"=w321, "integral time (Ti, min)"=w320, "derivative time (Td, min)"=w319) -> (w322:T5)
            n112 = Not Equal?(x=w310, y=w326) -> (x != y?=w325:bool)
            n113 = First Call?() -> (First Call?: T/F=w318:bool)
            n114 = Bundle By Name(cluster=cluster{"setpoint high":dbl, "setpoint low":dbl} {"setpoint high"=100.0, "setpoint low"=0.0} ("setpoint range"), "setpoint high"=w312, "setpoint low"=w313) -> (w307:cluster{"setpoint high":dbl, "setpoint low":dbl})
            n115 = Or(x=w325, y=w318) -> (x .or. y?=w324:bool)
            n116 = call-poly <vilib>:"PID Advanced.vi"("setpoint"=w308, "output range"=cluster{"output high":dbl, "output low":dbl} {"output high"=100.0, "output low"=0.0}, "auto? (T)"=w309, "manual control"=w308, "process variable"=w328, "setpoint range"=w307, "PID gains"=w322, "reinitialize? (F)"=w324) -> ("output"=w316:dbl)  [unwired: 6 in, 1 out]
            n117 = call "Set Output Pct.vi"("Output %"=w316, "Pump in"=w317) -> ()  [unwired: 8 in, 2 out]
            n118 = call <vilib>:"Add State(s) to Queue__jki_lib_state_machine.vi"("State(s) in (\"\")"=w333) -> ("States Out"=w332:string)  [unwired: 14 in]
          }
          frame "Action: Read Speed" {
            n119 = Unbundle By Name(w348) -> ("Self Reference"=w336:refnum<class "Pump.lvclass">)
            n120 = call-dynamic "readPumpSpeed.vi"("Pump in"=w336) -> ("error out"=w344:errorcluster, "Pump Speed"=w345:dbl, "Pump out"=w339:refnum<class "Pump.lvclass">)  [unwired: 8 in]
            n121 = call-dynamic "Get Output Pct.vi"("Pump in"=w336) -> ("error out"=w334:errorcluster, "Output %"=w335:dbl)  [unwired: 8 in, 1 out]
            n122 = call "Get Setpoint.vi"("Pump in"=w336) -> ("error out"=w343:errorcluster, "Pump Setpoint"=w346:dbl)  [unwired: 8 in, 1 out]
            n123 = Bundle By Name(cluster=w348, "Speed"=w345) -> (w347:T7)
            n124 = Bundle(cluster=T1 {"Pump Setpoint"=0.0, "Pump Speed"=0.0, "Output %"=0.0} ("Pump State"), "Pump Setpoint"=w346, "Pump Speed"=w345, "Output %"=w335) -> (w338:T1)
            "Pump State" <- w338
            n125 = call "Generate Pump State Event.vi"("Pump State"=w338, "Pump in"=w339) -> ("error out"=w337:errorcluster)  [unwired: 8 in, 1 out]
            n126 = Merge Errors(w342, w344, w343, w337, w334) -> (w341:errorcluster)
            n127 = call <vilib>:"Add State(s) to Queue__jki_lib_state_machine.vi"("State(s) in (\"\")"=w351) -> ("States Out"=w350:string)  [unwired: 14 in]
          }
        }
      }
    }
    frame Error {
    }
  }
  n128 = call-parent "Process.vi"("error in"=w10, "SMO"=w9) -> ("error out"=w8:errorcluster, "SMO out"=→"Pump out":refnum<class "Pump.lvclass">)  [unwired: 8 in]
  n129 = Merge Errors(w8, w7) -> (→"error out":errorcluster)
